vi "test.OutputReader.vi"(8 "error in":errorcluster, 10 "Buffer in":string, 11 "Variant":variant) -> (0 "error out":errorcluster)   [LabVIEW 2014]
panel:
  out "out":string
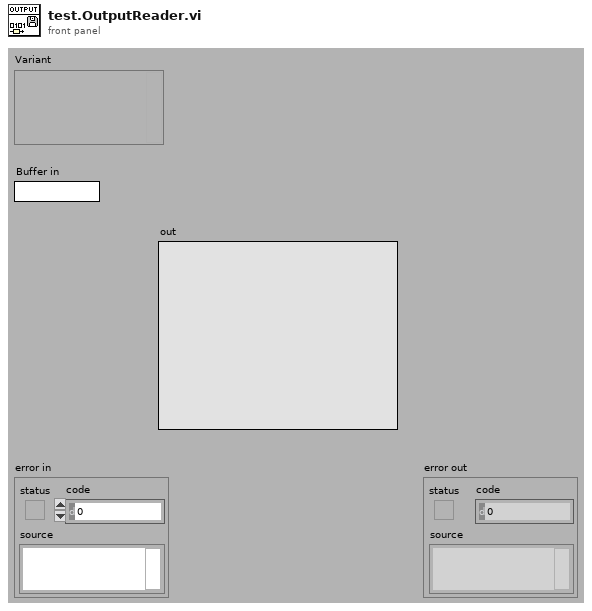
[diagram p1: front panel]
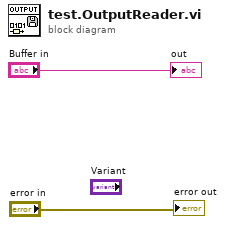
[diagram p0: block diagram]
diagram:
  "error out" <- "error in"
  "out" <- "Buffer in"
